vi "New Execution.vi"(8 "error in (no error)":errorcluster, 10 "Execution Options":T1, 11 "Engine in":refnum<class "Engine.lvclass">) -> (0 "error out":errorcluster, 2 "Execution":refnum<class "Execution.lvclass">, 3 "Engine out":refnum<class "Engine.lvclass">)   [LabVIEW 2020, in "TSnax.lvlib" / "Engine.lvclass"]
uses:
  Engine.lvclass
  Execution/Execution Options.ctl
  Execution/Execution.lvclass
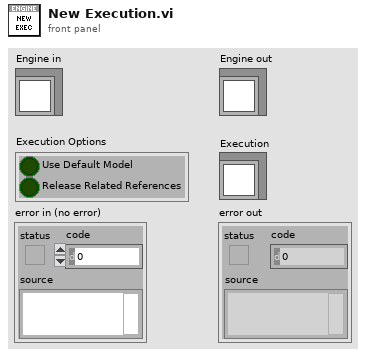
[diagram p1: front panel]
types:
  T1 = typedef "TSnax.lvlib/Execution.lvclass/Execution Options.ctl" = cluster{"Use Default Model":bool, "Release Related References":bool}
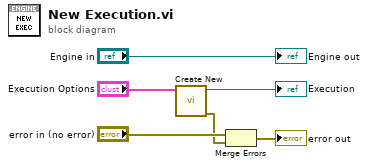
[diagram p0: block diagram]
diagram:
  n1 = call "Create New.vi"("Options"="Execution Options") -> ("error out"=w1:errorcluster, "Execution out"=→"Execution":refnum<class "Execution.lvclass">)  [unwired: 9 in]
  n2 = Merge Errors("error in (no error)", w1) -> (→"error out":errorcluster)
  "Engine out" <- "Engine in"
